vi "Create Unique Queue.vi"(8 "error in (no error)":errorcluster) -> (0 "error out":errorcluster, 3 "Queue out":refnum<class "Queue.lvclass">)   [LabVIEW 2013, in "Architecture.lvlib" / "Queue.lvclass"]
uses:
  Queue.lvclass
  Message.lvclass
  Queue.lvclass/Queue.ctl
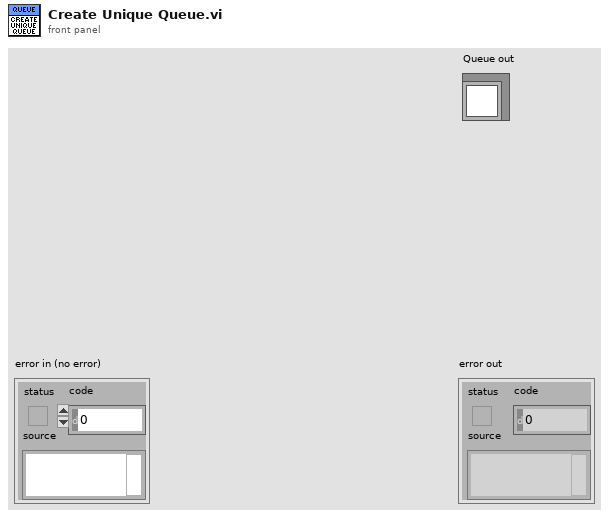
[diagram p1: front panel]
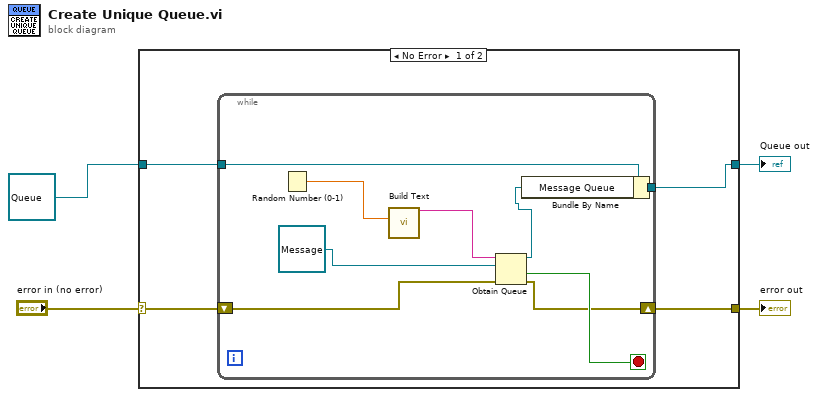
[diagram p0: block diagram]
diagram:
  n1 = case shown="No Error" "error in (no error)" {
    selector: "error in (no error)" -> [w7 w19]
    tunnel: [w6 w19] -> w3
    tunnel: [w5 w18] -> w1
    tunnel: refnum<class "Queue.lvclass"> refnum ("Queue in") -> [w8 w18]
    frame No Error {
      n2 = while {
        tunnel: w8 -> [w11]
        shift-right: [w12] -> w6
        shift-left: w7 -> [w14]
        tunnel: [w9] -> w5
        stop <- w13 stop-if-true
        n3 = Random Number (0-1)() -> (number: 0 to 1=w17:dbl)
        n4 = call "Build Text"("random"=w17) -> ("Result"=w15:string)  [unwired: 13 in, 1 out]
        n5 = Obtain Queue(name (unnamed)=w15, element data type=refnum<class "Message.lvclass"> refnum ("Architecture.lvlib:Message.lvclass"), error in (no error)=w14) -> (queue out=w10:refnum<queue>, created new?=w13:bool, error out=w12:errorcluster)  [unwired: 2 in]
        n6 = Bundle By Name(cluster=w11, "Message Queue"=w10) -> (w9:refnum<class "Queue.lvclass">)
      }
    }
    frame Error {
    }
  }
  "error out" <- w3
  "Queue out" <- w1
